vi "encode varint.vi"(11 "value":u64) -> (3 "byte array out":u8[](array[numeric]) format="%.0b")   [LabVIEW 2013, in "protocol buffers encoder.lvlib"]
uses:
  protocol buffers encoder.lvlib
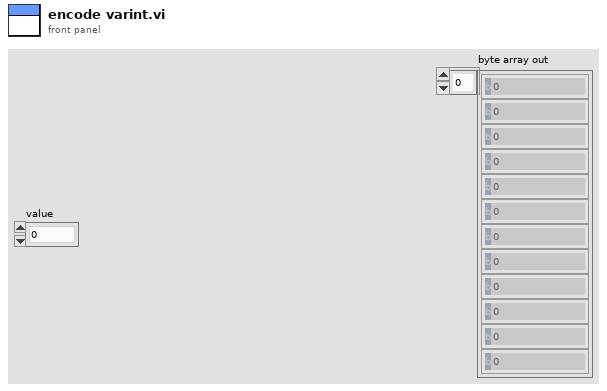
[diagram p1: front panel]
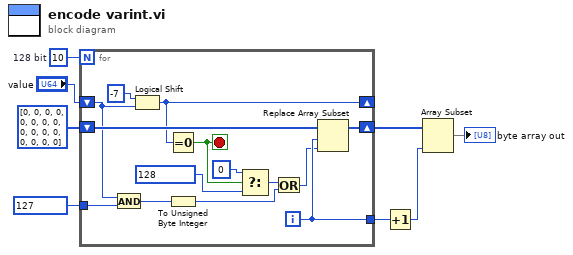
[diagram p0: block diagram]
diagram:
  w8 = 10  # 128 bit
  n1 = for {
    N: w8 -> [_]
    shift-right: [w20] -> w4
    shift-left: u8[] [0, 0, 0, 0, 0, 0, 0, 0, 0, 0, 0, 0, 0, 0, 0, 0] -> [w21]
    shift-right: [w17] -> _
    shift-left: "value" -> [w14]
    tunnel: [w19] -> w5
    tunnel: u8 127 -> [w22]
    i -> [w19]
    stop <- w16 stop-if-true
    n2 = And(x=w14, y=w22) -> (x .and. y?=w15:u64)
    n3 = Logical Shift(y=i16 -7, x=w14) -> (x << y=w17:u64)
    n4 = Equal To 0?(x=w17) -> (x = 0?=w16:bool)
    n5 = To Unsigned Byte Integer(number=w15) -> (unsigned 8bit integer=w12:u8)
    n6 = Select(t=u8 0, s=w16, f=u8 128) -> (s? t:f=w13:u8)
    n7 = Or(x=w13, y=w12) -> (x .or. y?=w11:u8)
    n8 = Replace Array Subset(array=w21, new element=w11, index=w19) -> (w20:u8[])
  }
  n9 = Increment(x=w5) -> (x+1=w3:i32)
  n10 = Array Subset(array=w4, length=w3) -> (→"byte array out":u8[])  [unwired: 1 in]
